vi "VI Server Control N2.vi"(0 "VI Server Control N2":T1={"VI name"="", "Control"=[], "Value"=[], "Boolean?"=[], "Wait Option"=enum."Wait Until", "wait (sec)"=0.0, "Control to End"="", "finish boolean?"=enum."boolean", "Condition"=enum."Boolean OFF", "Target Value"=120.0, "xxx%"=120.0, "update every (s)"=120.0, "Timeout (sec)"=10000.0} {"Boolean?" min=0.0 max=1.0 step=1.0 format="%#_1g"}) -> ()   [LabVIEW 2020]
uses:
  Units/VI Server Control N2/VI Server Control N2.ctl
  Units/VI Server Control N2/condition.ctl
panel:
  out "initial value":dbl
  out "error out":errorcluster
  # "Value of Control\n(if control is boolean type\n1 for \"ON\" and,0 for \"OFF\")"
  # "Is this control Boolean?\n(Yes: 1,  No: 0)"
  # "Name of  Control"
  # "0"
  # "1"
  # "2"
  # "3"
  # "4"
  # "5"
  # "6"
  # "7"
  # "8"
  # "9"
  # "1."
  # "Purely wait for"
  # "seconds"
  # "Control / Indicator Name"
  # "2."
  # "which is"
  # "Finish if"
  # "meets the following conditions"
  # "(check and update every"
  # "seconds)"
  # "3. Timeout"
  # "and also finish the whole thing if time elapses"
  # "or longer."
  # "Wait until the following condition meets."
  # "Do not wait and move on to the next line in sequence."
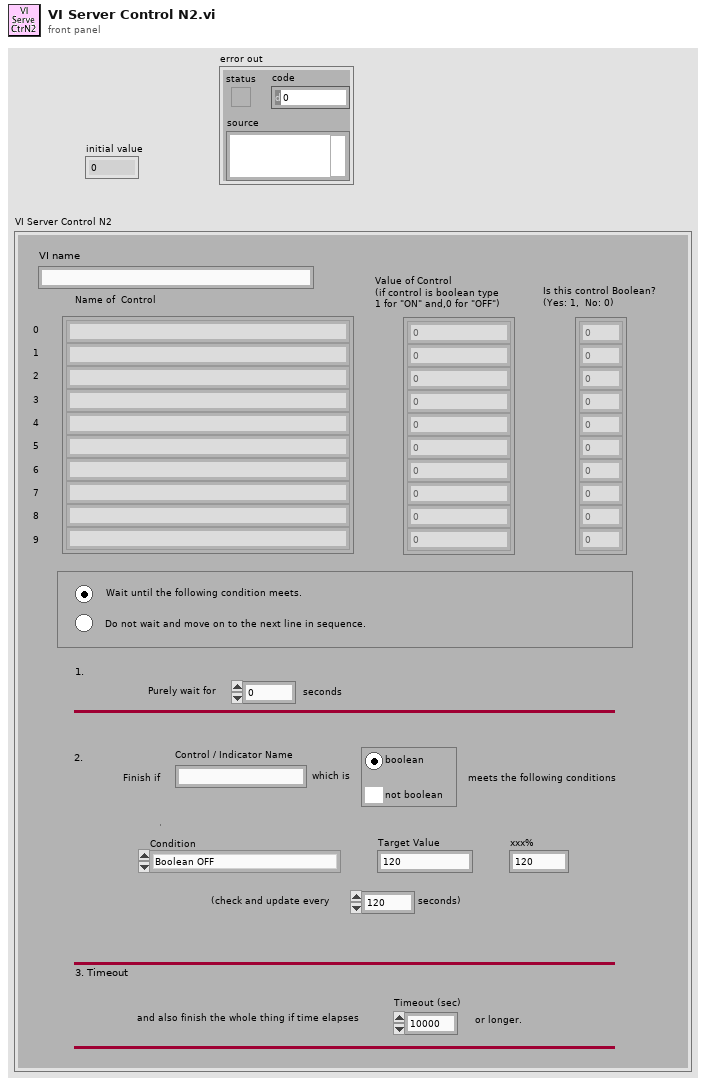
[diagram p1: front panel]
types:
  T1 = typedef "VI Server Control N2.ctl" = cluster{"VI name":string, "Control":string[], "Value":dbl[], "Boolean?":dbl[], "Wait Option":enum32{"Wait Until", "Do Not Wait"}, "wait (sec)":dbl, "Control to End":string, "finish boolean?":enum32{"boolean", "not boolean"}, "Condition":T2, "Target Value":dbl, "xxx%":dbl, "update every (s)":dbl, "Timeout (sec)":dbl}
  T2 = typedef "condition.ctl" = enum16{"within xxx% of target value", "<= target value", ">= target value", "= target value", "Boolean ON", "Boolean OFF"}
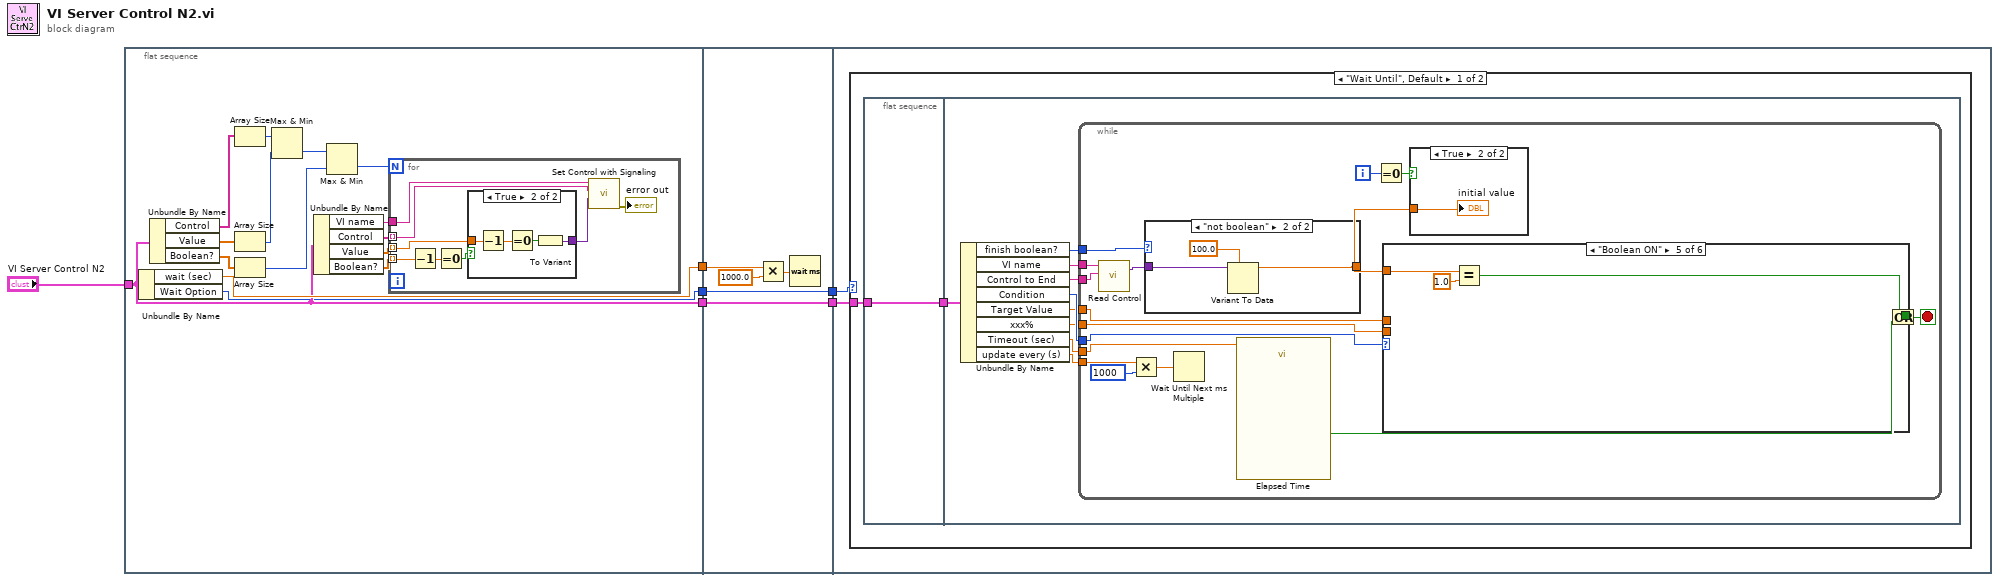
[diagram p0: block diagram]
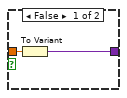
[diagram p2: hidden frame]
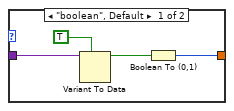
[diagram p4: hidden frame]
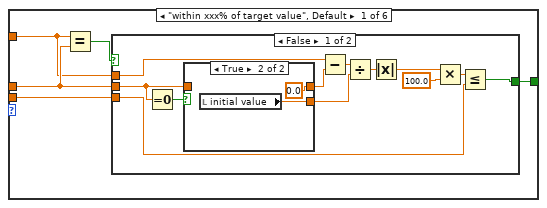
[diagram p5: hidden frame]
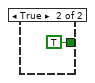
[diagram p7: hidden frame]
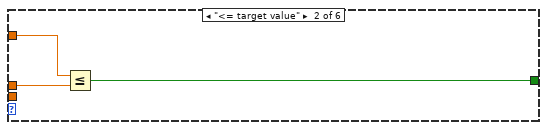
[diagram p8: hidden frame]
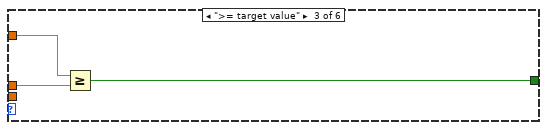
[diagram p9: hidden frame]
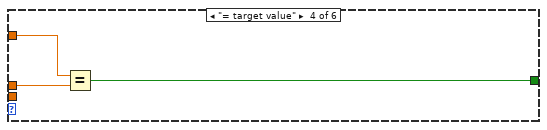
[diagram p10: hidden frame]
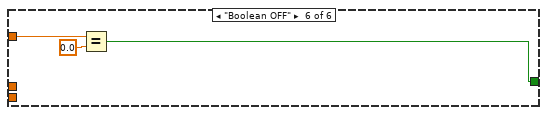
[diagram p11: hidden frame]
diagram:
  n1 = flat-sequence {
    tunnel: "VI Server Control N2" -> [w8]
    tunnel: [w9] -> w5
    tunnel: [w8] -> w3
    tunnel: [w7] -> w1
    tunnel: w5 -> [w36]
    tunnel: [w39] -> w4
    tunnel: w3 -> [w39]
    tunnel: [w40] -> w2
    tunnel: w1 -> [w40]
    tunnel: w4 -> [w42]
    tunnel: w2 -> [w41]
    frame #0 {
      n2 = Unbundle By Name(w8) -> ("wait (sec)"=w9:dbl, "Wait Option"=w7:enum32{"Wait Until", "Do Not Wait"})
      n3 = Unbundle By Name(w8) -> ("Control"=w21:string[], "Value"=w20:dbl[], "Boolean?"=w14:dbl[])
      n4 = Array Size(array=w21) -> (size(s)=w19:i32)
      n5 = Array Size(array=w20) -> (size(s)=w18:i32)
      n6 = Array Size(array=w14) -> (size(s)=w16:i32)
      n7 = Max & Min(x=w19, y=w18) -> (min(x,y)=w17:i32)  [unwired: 1 out]
      n8 = Unbundle By Name(w8) -> ("VI name"=w11:string, "Control"=w10:string[], "Value"=w12:dbl[], "Boolean?"=w13:dbl[])
      n9 = Max & Min(x=w17, y=w16) -> (min(x,y)=w15:i32)  [unwired: 1 out]
      n10 = for {
        N: w15 -> [_]
        tunnel: w13 -> [w29] mode=indexing
        tunnel: w12 -> [w26] mode=indexing
        tunnel: w11 -> [w25]
        tunnel: w10 -> [w23] mode=indexing
        n11 = Decrement(x=w29) -> (x-1=w28:dbl)
        n12 = Equal To 0?(x=w28) -> (x = 0?=w27:bool)
        n13 = case shown="True" w27 {
          tunnel: w26 -> [w30 w34]
          tunnel: [w31 w33] -> w24
          frame False {
            n14 = To Variant(anything=w30) -> (Variant=w31:variant)
          }
          frame True {
            n15 = Decrement(x=w34) -> (x-1=w35:dbl)
            n16 = Equal To 0?(x=w35) -> (x = 0?=w32:bool)
            n17 = To Variant(anything=w32) -> (Variant=w33:variant)
          }
        }
        n18 = call "Set Control with Signaling.vi"("Value"=w24, "Control Name"=w23, "VI Name"=w25) -> ("error out"=→"error out":errorcluster)  [unwired: 8 in]
      }
    }
    frame #1 {
      n19 = Multiply(x=w36, y=1000.0) -> (x*y=w38:dbl)
      n20 = Wait (ms)(milliseconds to wait=w38) -> ()  [unwired: 1 out]
    }
    frame #2 {
      n21 = case shown="\"Wait Until\", Default" w41 {
        tunnel: w42 -> [w44 _]
        frame "Wait Until", Default {
          n22 = flat-sequence {
            tunnel: w44 -> [w45]
            tunnel: [w45] -> w43
            tunnel: w43 -> [w54]
            frame #0 {
            }
            frame #1 {
              n23 = Unbundle By Name(w54) -> ("finish boolean?"=w46:enum32{"boolean", "not boolean"}, "VI name"=w53:string, "Control to End"=w52:string, "Condition"=w51:T2, "Target Value"=w50:dbl, "xxx%"=w49:dbl, "Timeout (sec)"=w48:dbl, "update every (s)"=w47:dbl)
              n24 = while {
                tunnel: w53 -> [w71]
                tunnel: w52 -> [w70]
                tunnel: w51 -> [w68]
                tunnel: w50 -> [w67]
                tunnel: w49 -> [w66]
                tunnel: w48 -> [w63]
                tunnel: w47 -> [w60]
                tunnel: w46 -> [w58]
                i -> [w57]
                stop <- w64 stop-if-true
                n25 = call "Read Control.vi"("VI Name"=w71, "Control Name"=w70) -> ("Value"=w69:variant)  [unwired: 3 in, 1 out]
                n26 = Multiply(x=w60, y=1000) -> (x*y=w59:dbl)
                n27 = case shown="\"not boolean\"" w58 {
                  tunnel: w69 -> [w76 w78]
                  tunnel: [w73 w77] -> w55
                  frame "boolean", Default {
                    n28 = Variant To Data(type=TRUE, Variant=w76) -> (data=w74:bool)  [unwired: 1 in, 1 out]
                    n29 = Boolean To (0,1)(Boolean=w74) -> (0, 1=w73:i16)
                  }
                  frame "not boolean" {
                    n30 = Variant To Data(type=100.0 ("y"), Variant=w78) -> (data=w77:dbl)  [unwired: 1 in, 1 out]
                  }
                }
                n31 = Wait Until Next ms Multiple(millisecond multiple=w59) -> ()  [unwired: 1 out]
                n32 = call "Elapsed Time"("Time Target (s)"=w63) -> ("Time has Elapsed"=w62:bool)  [unwired: 11 in, 7 out]
                n33 = Equal To 0?(x=w57) -> (x = 0?=w56:bool)
                n34 = case shown="\"Boolean ON\"" w68 {
                  tunnel: w67 -> [w82 w101 w104 w107 _ _]
                  tunnel: [w83 w103 w106 w109 w110 w113] -> w65
                  tunnel: w66 -> [w81 _ _ _ _ _]
                  tunnel: w55 -> [w80 w102 w105 w108 w112 w114]
                  frame "within xxx% of target value", Default {
                    n35 = Equal?(x=w80, y=w82) -> (x = y?=w84:bool)
                    n36 = case shown="False" w84 {
                      tunnel: [w88 TRUE] -> w83
                      tunnel: w82 -> [w91 _]
                      tunnel: w81 -> [w92 _]
                      tunnel: w80 -> [w85 _]
                      frame False {
                        n37 = Equal To 0?(x=w91) -> (x = 0?=w96:bool)
                        n38 = case shown="True" w96 {
                          tunnel: [w97 0.0 ("Target Value")] -> w87
                          tunnel: w91 -> [w97 _]
                          tunnel: [w97 w98] -> w86
                          frame False {
                          }
                          frame True {
                            n39 = local read "initial value"() -> (w98:dbl)
                          }
                        }
                        n40 = Subtract(x=w85, y=w87) -> (x-y=w89:dbl)
                        n41 = Divide(x=w89, y=w86) -> (x/y=w90:dbl)
                        n42 = Absolute Value(x=w90) -> (abs(x)=w93:dbl)
                        n43 = Multiply(x=w93, y=100.0) -> (x*y=w94:dbl)
                        n44 = Less Or Equal?(x=w94, y=w92) -> (x <= y?=w88:bool)
                      }
                      frame True {
                      }
                    }
                  }
                  frame "<= target value" {
                    n45 = Less Or Equal?(x=w102, y=w101) -> (x <= y?=w103:bool)
                  }
                  frame ">= target value" {
                    n46 = Greater Or Equal?(x=w105, y=w104) -> (x >= y?=w106:bool)
                  }
                  frame "= target value" {
                    n47 = Equal?(x=w108, y=w107) -> (x = y?=w109:bool)
                  }
                  frame "Boolean ON" {
                    n48 = Equal?(x=w112, y=1.0) -> (x = y?=w110:bool)
                  }
                  frame "Boolean OFF" {
                    n49 = Equal?(x=w114, y=0.0) -> (x = y?=w113:bool)
                  }
                }
                n50 = case shown="True" w56 {
                  tunnel: w55 -> [_ w72]
                  frame False {
                  }
                  frame True {
                    "initial value" <- w72
                  }
                }
                n51 = Or(x=w65, y=w62) -> (x .or. y?=w64:bool)
              }
            }
          }
        }
        frame "Do Not Wait" {
        }
      }
    }
  }
